vi "RT Main.vi"   [LabVIEW 2013]
doc: "本模板用于队列消息处理器设计模式。\n\n事件处理循环负责按用户界面操作生成对应的消息。\n\n消息处理循环负责对事件处理循环或其他消息生成的消息进行处理。消息内容为字符串值，因此很容易将新消息添加至“消息处理”循环的“消息分支”条件结构。每个消息簇还可选择性地为消息数据提供一个变体，变体数据可以转换为消息数据所需要的任意类型。"
uses:
  Globals/Global - All RT Loop Stop.vi
  Globals/Global - Configuration Options.vi
  Globals/Global - Monitoring Variables.vi
  Globals/Global - RT Stream Connections.vi
  support/Message Queue/Message Queue.lvlib
  <vilib>/nisyscfg/nisyscfg.lvlib
types:
  T1 = typedef "Acquisition and Logging Configuration.ctl" = cluster{"Data Rate (Hz)":dbl, "Samples per Read":i32, "Number of Reads to Save":i32, "Data File Name":string, "TDMS Properties":T2[], "Number of Channels":i32, "Channel Scale Array":dbl[], "Channel Names":string[], "Trigger - RMS Value":dbl, "Trigger - Channel":i32, "Trigger - Time (Minute)":i32, "Enable RMS Trigger":bool, "Enable Time Trigger":bool, "Always Log":bool}
  T2 = typedef "TDMS Properties.ctl" = cluster{"Name":string, "Value":string}
  T3 = typedef "Message Queue.lvlib/All Real-Time Message Queues.ctl" = cluster{"Message Handler":refnum<queue>, "Acquisition and Logging":refnum<queue>}
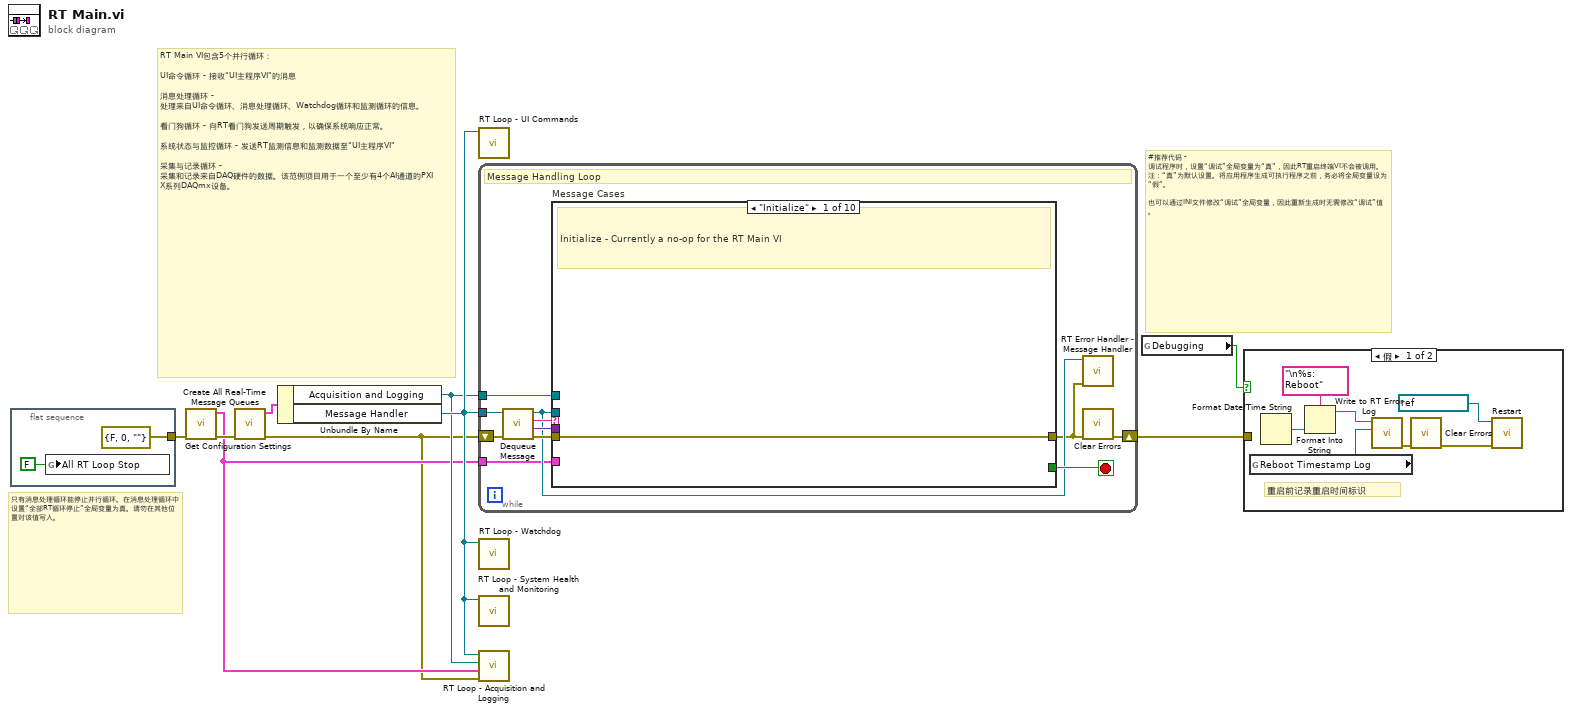
[diagram p0: block diagram]
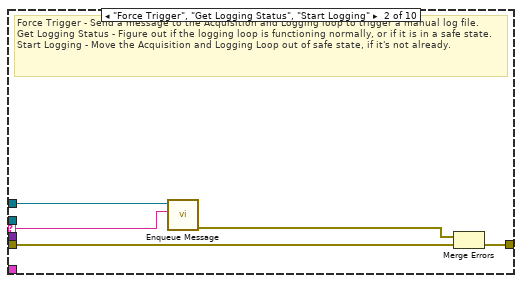
[diagram p3: hidden frame]
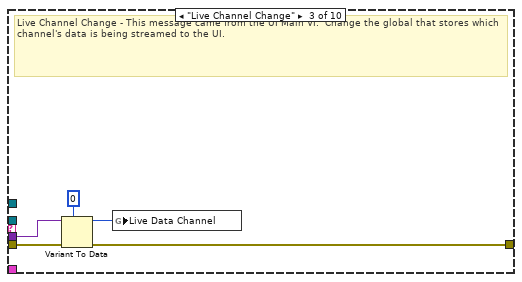
[diagram p4: hidden frame]
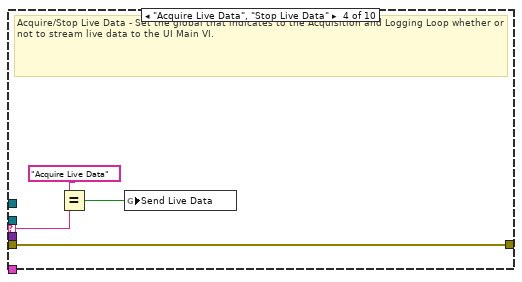
[diagram p5: hidden frame]
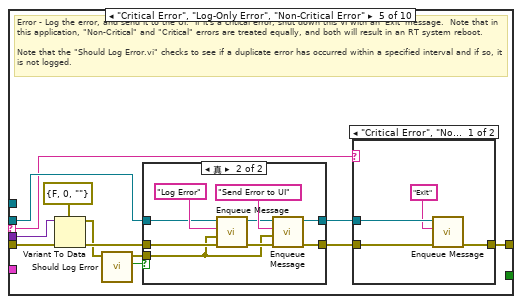
[diagram p6: hidden frame]
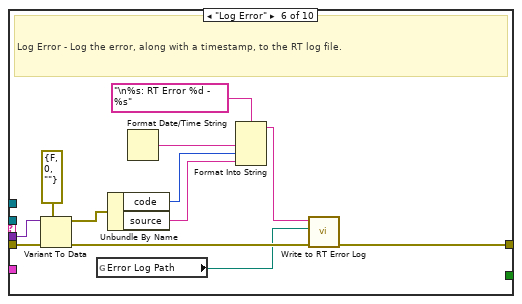
[diagram p9: hidden frame]
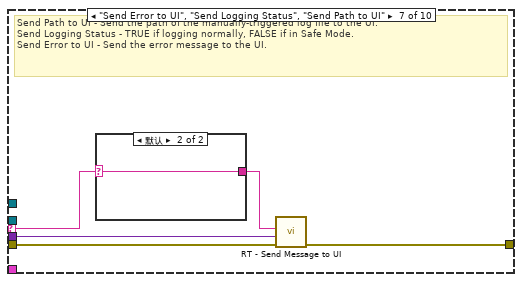
[diagram p10: hidden frame]
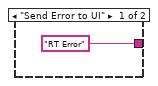
[diagram p11: hidden frame]
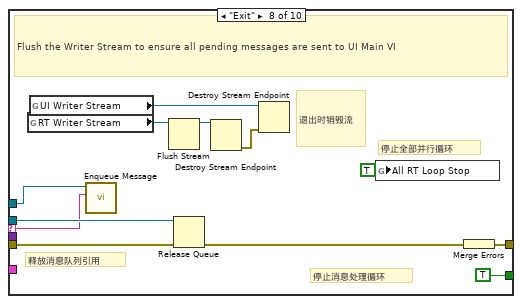
[diagram p12: hidden frame]
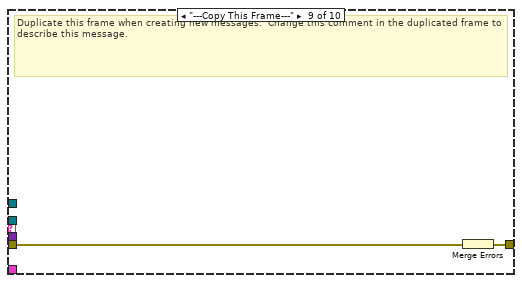
[diagram p13: hidden frame]
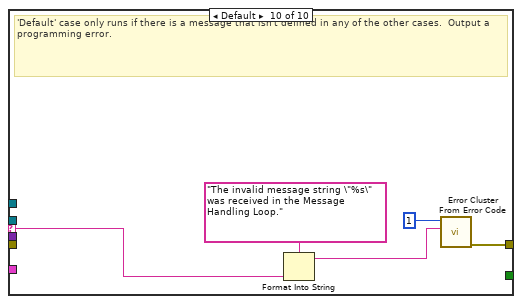
[diagram p14: hidden frame]
diagram:
  # "#推荐代码 - 调试程序时，设置“调试”全局变量为“真”，因此RT重启终端VI不会被调用。注：“真”为默认设置。将应用程序生成可执行程序之前，务必将全局变量设为“假”。\n\n也可以通过INI文件修改“调试”全局变量，因此重新生成时无需修改“调试”值。"
  # "RT Main VI包含5个并行循环：\n\nUI命令循环 - 接收\"UI主程序VI\"的消息\n\n消息处理循环 - 处理来自UI命令循环、消息处理循环、Watchdog循环和监测循环的信息。\n\n看门狗循环 - 向RT看门狗发送周期触发，以确保系统响应正常。\n\n系统状态与监控循环 - 发送RT监测信息和监测数据至\"UI主程序VI\"\n\n采集与记录循环 - 采集和记录来自DAQ硬件的数据。该范例项目用于一个至少有4个AI通道的PXI X系列DAQmx设备。"
  # "只有消息处理循环能停止并行循环。在消息处理循环中设置“全部RT循环停止”全局变量为真。请勿在其他位置对该值写入。"
  n1 = flat-sequence {
    tunnel: [errorcluster {"status"=FALSE, "code"=0, "source"=""} ("error constant")] -> w9
    frame #0 {
      n2 = global write "Global - All RT Loop Stop.vi" "All RT Loop Stop"(FALSE) -> ()
    }
  }
  n3 = call "Get Configuration Settings.vi"("error in (no error)"=w9) -> ("error out"=w6:errorcluster, "Acquisition and Logging Configuration"=w2:T1)  [unwired: 9 in]
  n4 = call "Create All Real-Time Message Queues.vi"("error in (no error)"=w6) -> ("error out"=w1:errorcluster, "Message Queues out"=w4:T3)  [unwired: 9 in]
  n5 = Unbundle By Name(w4) -> ("Acquisition and Logging"=w3:refnum<queue>, "Message Handler"=w5:refnum<queue>)
  n6 = call "RT Loop - UI Commands.vi"("Message Queue"=w5) -> ()  [unwired: 11 in]
  n7 = while {
    tunnel: w5 -> [w17]
    shift-right: [w15] -> w8
    shift-left: w1 -> [w21]
    tunnel: w3 -> [w13]
    tunnel: w2 -> [w12]
    stop <- w22 stop-if-true
    # "Message Handling Loop"
    n8 = call "Dequeue Message.vi"("error in (no error)"=w21, "Message Queue"=w17) -> ("error out"=w20:errorcluster, "Message Data"=w18:variant, "Message"=w19:string, "dup Message Queue"=w16:refnum<queue>)  [unwired: 6 in]
    n9 = case "Message Cases" shown="\"Initialize\"" w19 {
      selector: w19 -> [_ w26 _ w36 w43 _ w79 w87 _ w102]
      tunnel: w16 -> [_ _ _ _ w44 _ _ w96 _ _]
      tunnel: w20 -> [w23 w28 w33 w37 w46 w77 w82 w92 w98 _]
      tunnel: [w23 w25 w32 w37 w49 w68 w81 w93 w97 w100] -> w14
      tunnel: [_ _ _ _ _ _ _ TRUE _ _] -> w22
      tunnel: w18 -> [_ _ w31 _ w38 w76 w80 _ _ _]
      tunnel: w13 -> [_ w27 _ _ _ _ _ w88 _ _]
      tunnel: w12 -> [_ _ _ _ _ _ _ _ _ _]
      frame "Initialize" {
        # "Initialize - Currently a no-op for the RT Main VI"
      }
      frame "Force Trigger", "Get Logging Status", "Start Logging" {
        # "Force Trigger - Send a message to the Acquisition and Logging loop to trigger a manual log file.\nGet Logging Status - Figure out if the logging loop is functioning normally, or if it is in a safe state.\nStart Logging - Move the Acquisition and Logging Loop out of safe state, if it's not already."
        n10 = call "Enqueue Message.vi"("Message"=w26, "Message Queue"=w27) -> ("error out"=w24:errorcluster)  [unwired: 8 in, 1 out]
        n11 = Merge Errors(w24, w28) -> (w25:errorcluster)
      }
      frame "Live Channel Change" {
        # "Live Channel Change - This message came from the UI Main VI.  Change the global that stores which channel's data is being streamed to the UI."
        n12 = Variant To Data(error in=w33, type=u32 0, Variant=w31) -> (data=w29:u32, error out=w32:errorcluster)
        n13 = global write "Global - Monitoring Variables.vi" "Live Data Channel"(w29) -> ()
      }
      frame "Acquire Live Data", "Stop Live Data" {
        # "Acquire/Stop Live Data - Set the global that indicates to the Acquisition and Logging Loop whether or not to stream live data to the UI Main VI."
        n14 = Equal?(x="Acquire Live Data", y=w36) -> (x = y?=w34:bool)
        n15 = global write "Global - Monitoring Variables.vi" "Send Live Data"(w34) -> ()
      }
      frame "Critical Error", "Log-Only Error", "Non-Critical Error" {
        # "Error - Log the error, and send it to the UI.  If it's a critical error, shut down this VI with an 'Exit' message.  Note that in this application, \"Non-Critical\" and \"Critical\" errors are treated equally, and both will result in an RT system reboot.\n\nNote that the \"Should Log Error.vi\" checks to see if a duplicate error has occurred within a specified interval and if so, it is not logged."
        n16 = Variant To Data(error in=w46, type=errorcluster {"status"=FALSE, "code"=0, "source"=""} ("error out"), Variant=w38) -> (data=w41:errorcluster, error out=w47:errorcluster)
        n17 = call "Should Log Error.vi"("error to report"=w41) -> ("Should Log Error?"=w39:bool, "dup error to report"=w40:errorcluster)  [unwired: 9 in]
        n18 = case shown="真" w39 {
          tunnel: [w51 w58] -> w45
          tunnel: [w50 w57] -> w42
          tunnel: w44 -> [w50 w56]
          tunnel: w47 -> [w51 w53]
          tunnel: w40 -> [_ w52]
          frame False {
          }
          frame True {
            n19 = call "Enqueue Message.vi"("error in (no error)"=w53, "Message Data"=w52, "Message"="Log Error", "Message Queue"=w56) -> ("error out"=w54:errorcluster, "dup Message Queue"=w55:refnum<queue>)  [unwired: 6 in]
            n20 = call "Enqueue Message.vi"("error in (no error)"=w54, "Message Data"=w52, "Message"="Send Error to UI", "Message Queue"=w55) -> ("error out"=w58:errorcluster, "dup Message Queue"=w57:refnum<queue>)  [unwired: 6 in]
          }
        }
        n21 = case shown="\"Critical Error\", \"Non-Critical Error\"" w43 {
          tunnel: w45 -> [w64 w65]
          tunnel: w42 -> [w62 _]
          tunnel: [w63 w65] -> w49
          frame "Critical Error", "Non-Critical Error" {
            n22 = call "Enqueue Message.vi"("error in (no error)"=w64, "Message"="Exit", "Message Queue"=w62) -> ("error out"=w63:errorcluster)  [unwired: 7 in, 1 out]
          }
          frame Default {
          }
        }
      }
      frame "Log Error" {
        # "Log Error - Log the error, along with a timestamp, to the RT log file."
        n23 = Variant To Data(error in=w77, type=errorcluster {"status"=FALSE, "code"=0, "source"=""} ("error constant"), Variant=w76) -> (data=w71:errorcluster, error out=w74:errorcluster)
        n24 = global read "Global - Configuration Options.vi" "Error Log Path"() -> (w66:path)
        n25 = Unbundle By Name(w71) -> ("code"=w70:i32, "source"=w69:string)
        n26 = Format Date/Time String() -> (date/time string=w72:string)  [unwired: 3 in]
        n27 = Format Into String(format string="\n%s: RT Error %d - %s", w72, w70, w69) -> (resulting string=w67:string)  [unwired: 2 in, 1 out]
        n28 = call "Write to RT Error Log.vi"("error in (no error)"=w74, "Error Log Path"=w66, "Log Entry"=w67) -> ("error out"=w68:errorcluster)  [unwired: 8 in]
      }
      frame "Send Error to UI", "Send Logging Status", "Send Path to UI" {
        # "Send Path to UI - Send the path of the manually-triggered log file to the UI.\nSend Logging Status - TRUE if logging normally, FALSE if in Safe Mode.\nSend Error to UI - Send the error message to the UI."
        n29 = case shown="默认" w79 {
          selector: w79 -> [_ w84]
          tunnel: ["RT Error" ("Message") w84] -> w78
          frame "Send Error to UI" {
          }
          frame Default {
          }
        }
        n30 = call "RT - Send Message to UI.vi"("error in (no error)"=w82, "Message Data"=w80, "Message"=w78) -> ("error out"=w81:errorcluster)  [unwired: 8 in]
      }
      frame "Exit" {
        # "退出时销毁流"
        # "停止消息处理循环"
        # "停止全部并行循环"
        # "释放消息队列引用"
        # "Flush the Writer Stream to ensure all pending messages are sent to UI Main VI"
        n31 = global read "Global - RT Stream Connections.vi" "RT Writer Stream"() -> (w86:refnum<k21>)
        n32 = global read "Global - RT Stream Connections.vi" "UI Writer Stream"() -> (w90:refnum<k21>)
        n33 = call "Enqueue Message.vi"("Message"=w87, "Message Queue"=w88) -> ()  [unwired: 8 in, 2 out]
        n34 = Flush Stream(11:w86) -> (3:w85:refnum<k21>)  [unwired: 3 in, 2 out]
        n35 = Release Queue(queue=w96, error in (no error)=w92) -> (error out=w94:errorcluster)  [unwired: 1 in, 2 out]
        n36 = Destroy Stream Endpoint(11:w85) -> (0:w89:errorcluster)  [unwired: 1 in]
        n37 = Destroy Stream Endpoint(8:w89, 11:w90) -> ()  [unwired: 1 out]
        n38 = global write "Global - All RT Loop Stop.vi" "All RT Loop Stop"(TRUE ("Stop Monitoring Loops")) -> ()
        n39 = Merge Errors(w94) -> (w93:errorcluster)
      }
      frame "---Copy This Frame---" {
        # "Duplicate this frame when creating new messages.  Change this comment in the duplicated frame to describe this message."
        n40 = Merge Errors(w98) -> (w97:errorcluster)
      }
      frame Default {
        # "'Default' case only runs if there is a message that isn't defined in any of the other cases.  Output a programming error."
        n41 = Format Into String(format string="The invalid message string \"%s\" was received in the Message Handling Loop." ("Unknown Message Error Text"), w102) -> (resulting string=w99:string)  [unwired: 2 in, 1 out]
        n42 = call <vilib>:"Error Cluster From Error Code.vi"("error message (\"\")"=w99, "error code (0)"=1) -> ("error out"=w100:errorcluster)  [unwired: 7 in]
      }
    }
    n43 = call "RT Error Handler - Message Handler.vi"("error in (no error)"=w14, "Message Queue"=w16) -> ()  [unwired: 9 in, 1 out]
    n44 = call <vilib>:"Clear Errors.vi"("error in (no error)"=w14) -> ("error out"=w15:errorcluster)  [unwired: 6 in]
  }
  n45 = call "RT Loop - Watchdog.vi"("Message Queue"=w5) -> ()  [unwired: 11 in]
  n46 = call "RT Loop - System Health and Monitoring.vi"("Message Queue"=w5) -> ()  [unwired: 11 in]
  n47 = call "RT Loop - Acquisition and Logging.vi"("error in (no error)"=w1, "Acquisition and Logging Configuration"=w2, "Acquisition and Logging Queue"=w3, "Message Queue"=w5) -> ()  [unwired: 8 in]
  n48 = global read "Global - Configuration Options.vi" "Debugging"() -> (w7:bool)
  n49 = case shown="假" w7 {
    tunnel: w8 -> [_ _]
    frame False {
      # "重启前记录重启时间标识"
      n50 = global read "Global - Configuration Options.vi" "Reboot Timestamp Log"() -> (w105:path)
      n51 = Format Date/Time String() -> (date/time string=w107:string)  [unwired: 3 in]
      n52 = Format Into String(format string="\n%s: Reboot", w107) -> (resulting string=w106:string)  [unwired: 2 in, 1 out]
      n53 = call "Write to RT Error Log.vi"("Error Log Path"=w105, "Log Entry"=w106) -> ("error out"=w110:errorcluster)  [unwired: 9 in]
      n54 = call <vilib>:"Clear Errors.vi"("error in (no error)"=w110) -> ("error out"=w109:errorcluster)  [unwired: 6 in]
      n55 = call <vilib>:"Restart.vi"("error in (no error)"=w109, "session in"=refnum<k21> "localhost") -> ()  [unwired: 7 in, 3 out]
    }
    frame True {
    }
  }
